vi "monitor.vi"() -> ()   [LabVIEW 2020]
panel:
  out "data_out":dbl[](array[numeric])
  out "controlled_end_point":bool
  in  "heading":dbl format="%.1f"
  in  "y":dbl=383827.29999999877 format="%.1f"
  in  "x":dbl=187655.50000000032 format="%.1f"
  out "XY Graph 2":cluster{"data_out":dbl[], "data_out":dbl[]}[](graph)
  out "endpoint_in_safetyarea":bool
  out "obstacle_in_safetyarea":bool
  out "XY Graph":cluster{"data_out":dbl[], "data_out":dbl[]}[](graph)
  in  "stop":bool
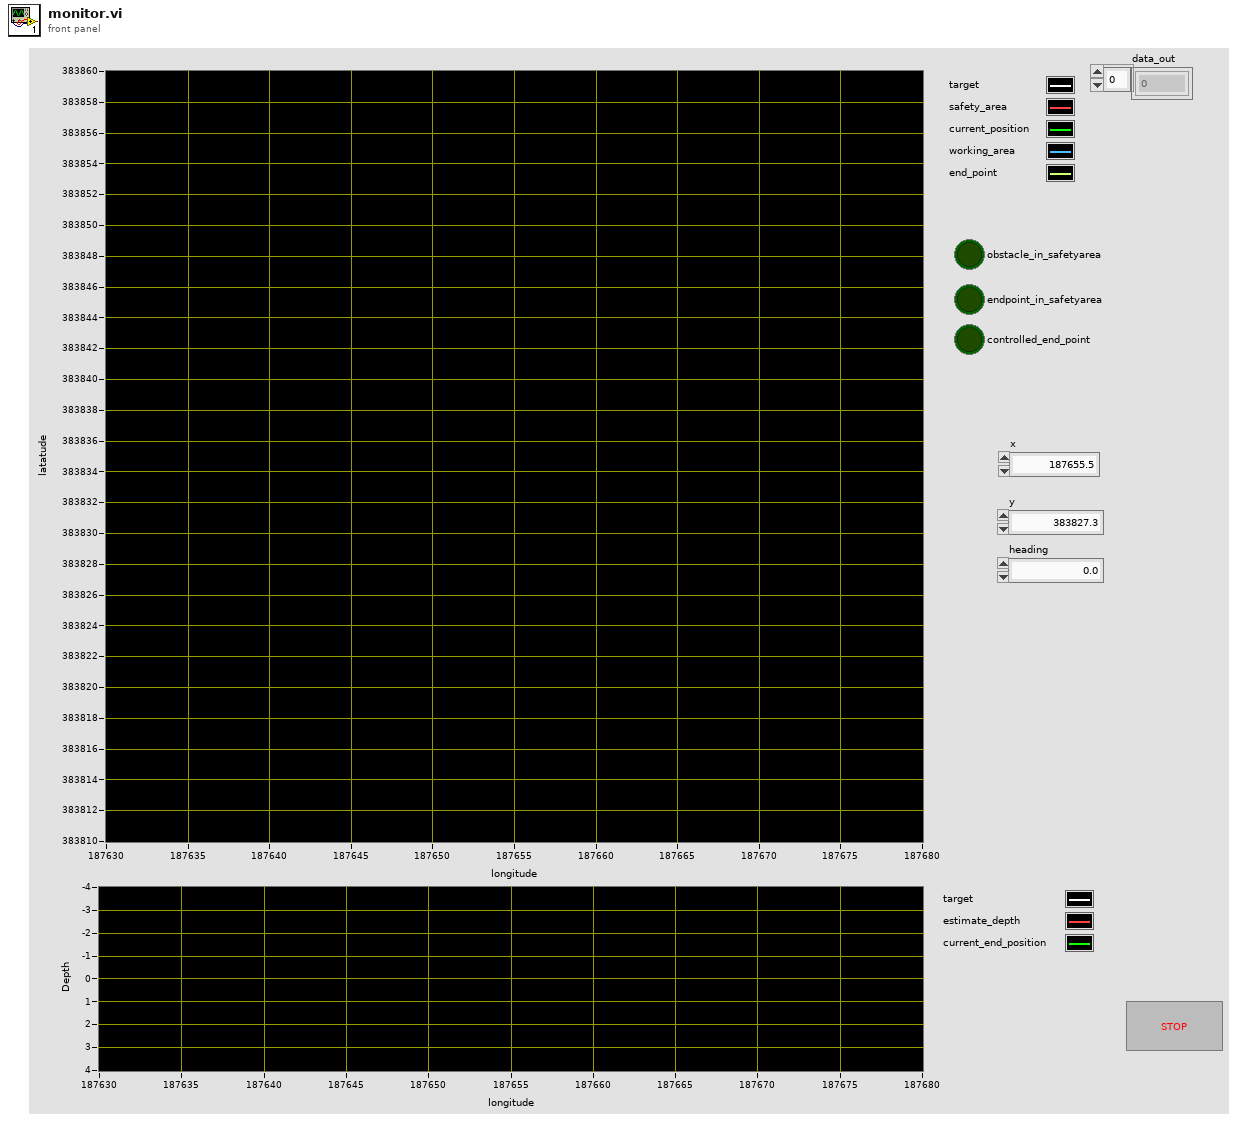
[diagram p1: front panel]
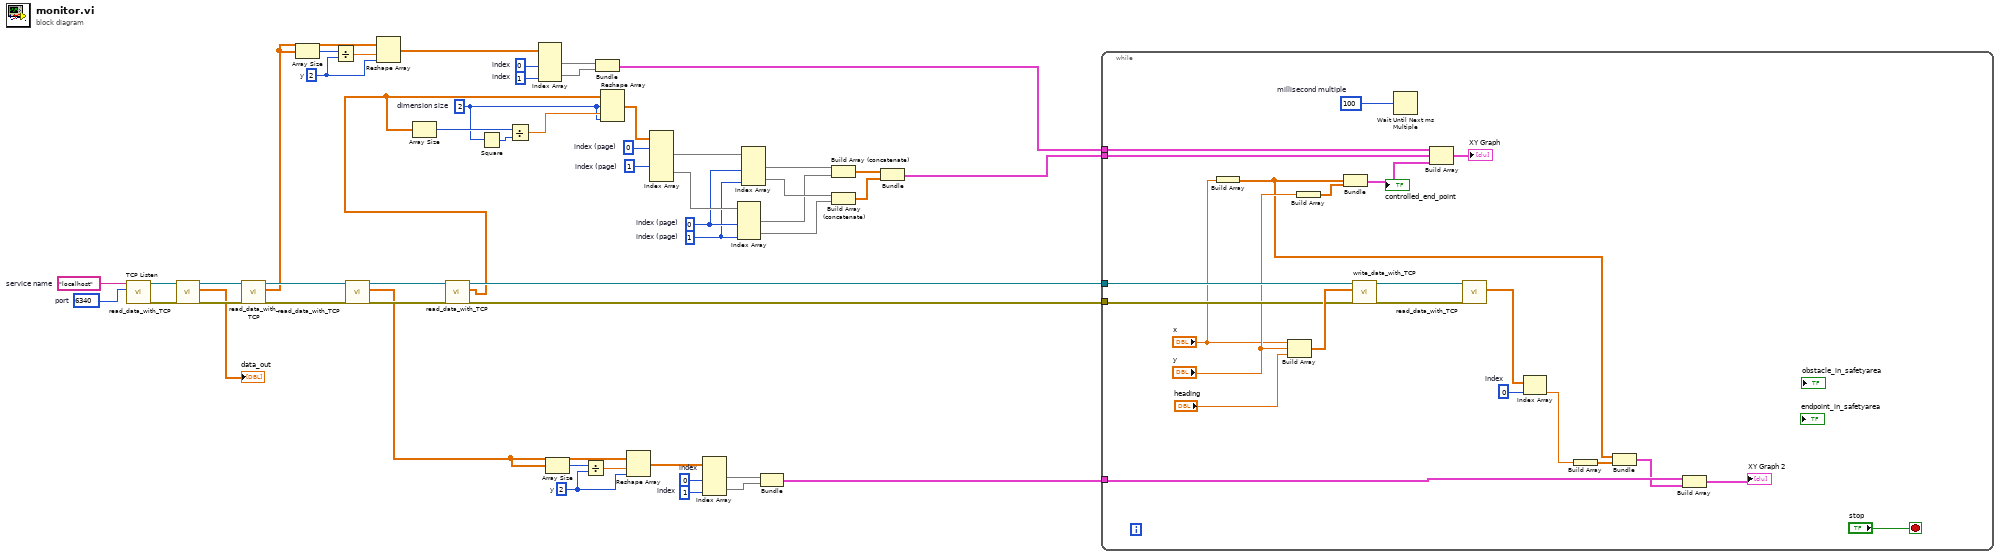
[diagram p0: block diagram]
diagram:
  w19 = 1  # index
  w18 = 0  # index
  w20 = 2  # y
  w25 = 1  # index (page)
  w27 = 1  # index (page)
  w28 = 0  # index (page)
  w26 = 0  # index (page)
  w29 = 2  # dimension size
  w45 = 1  # index
  w46 = 0  # index
  w44 = 2  # y
  w51 = u16 6340  # port
  w52 = "localhost"  # service name
  n1 = call <vilib>:"TCP Listen.vi"("port"=w51, "service name"=w52) -> ("error out"=w3:errorcluster, "connection ID"=w5:refnum<k5>)  [unwired: 5 in, 3 out]
  n2 = call "read_data_with_TCP.vi"("error_in"=w3, "TCP_ref_in"=w5) -> ("error_out"=w2:errorcluster, "data_out"=→"data_out":dbl[], "TCP_ref_out"=w4:refnum<k5>)  [unwired: 7 in]
  n3 = call "read_data_with_TCP.vi"("error_in"=w2, "TCP_ref_in"=w4) -> ("error_out"=w49:errorcluster, "data_out"=w43:dbl[], "TCP_ref_out"=w50:refnum<k5>)  [unwired: 7 in]
  n4 = Array Size(array=w43) -> (size(s)=w47:i32)
  n5 = Divide(x=w47, y=w44) -> (x/y=w48:dbl)
  n6 = call "read_data_with_TCP.vi"("error_in"=w49, "TCP_ref_in"=w50) -> ("error_out"=w14:errorcluster, "data_out"=w7:dbl[], "TCP_ref_out"=w15:refnum<k5>)  [unwired: 7 in]
  n7 = Reshape Array "Reshape Array"(w43, w48, w44) -> (w10:dbl[][])
  n8 = call "read_data_with_TCP.vi"("error_in"=w14, "TCP_ref_in"=w15) -> ("error_out"=w8:errorcluster, "data_out"=w6:dbl[], "TCP_ref_out"=w9:refnum<k5>)  [unwired: 7 in]
  n9 = Array Size(array=w6) -> (size(s)=w32:i32)
  n10 = Square(x=w29) -> (x^2=w33:i32)
  n11 = Divide(x=w32, y=w33) -> (x/y=w34:dbl)
  n12 = Index Array(array=w10, index (col) #1=w46, index (col) #2=w45) -> (element #1=w42:dbl[], element #2=w41:dbl[])  [unwired: 2 in]
  n13 = Array Size(array=w7) -> (size(s)=w17:i32)
  n14 = Divide(x=w17, y=w20) -> (x/y=w16:dbl)
  n15 = Bundle("data_out"=w42, "data_out"=w41) -> (w23:cluster{"data_out":dbl[], "data_out":dbl[]})  [unwired: 1 in]
  n16 = Reshape Array(w6, w29, w34, w29) -> (w30:dbl[][][])
  n17 = Reshape Array "Reshape Array"(w7, w16, w20) -> (w12:dbl[][])
  n18 = Index Array(array=w30, index (dim 0) #1=w26, index (dim 0) #2=w25) -> (element #1=w11:dbl[][], element #2=w31:dbl[][])  [unwired: 4 in]
  n19 = Index Array(array=w12, index (col) #1=w18, index (col) #2=w19) -> (element #1=w21:dbl[], element #2=w22:dbl[])  [unwired: 2 in]
  n20 = Index Array(array=w31, index (col) #1=w28, index (col) #2=w27) -> (element #1=w36:dbl[], element #2=w39:dbl[])  [unwired: 2 in]
  n21 = Index Array(array=w11, index (col) #1=w28, index (col) #2=w27) -> (element #1=w35:dbl[], element #2=w38:dbl[])  [unwired: 2 in]
  n22 = Bundle("data_out"=w21, "data_out"=w22) -> (w13:cluster{"data_out":dbl[], "data_out":dbl[]})  [unwired: 1 in]
  n23 = Build Array (concatenate)(w35, w36) -> (w37:dbl[])
  n24 = Build Array (concatenate)(w38, w39) -> (w40:dbl[])
  n25 = Bundle(w37, w40) -> (w24:cluster{dbl[], dbl[]})  [unwired: 1 in]
  n26 = while {
    tunnel: w24 -> [w72]
    tunnel: w23 -> [w73]
    tunnel: w13 -> [w61]
    tunnel: w9 -> [w70]
    tunnel: w8 -> [w69]
    stop <- "stop" stop-if-true
    w59 = 0  # index
    w68 = u32 100  # millisecond multiple
    n27 = Build Array("x") -> (w55:dbl[])
    n28 = Build Array("x", "y", "heading") -> (w71:dbl[])
    n29 = Build Array("y") -> (w63:dbl[])
    n30 = Bundle(w55, w63) -> (w62:cluster{dbl[], dbl[]})  [unwired: 1 in]
    n31 = call "write_data_with_TCP.vi"("error_in"=w69, "data_in"=w71, "TCP_ref_in"=w70) -> ("error_out"=w65:errorcluster, "TCP_ref_out"=w66:refnum<k5>)  [unwired: 7 in]
    n32 = Wait Until Next ms Multiple(millisecond multiple=w68) -> ()  [unwired: 1 out]
    n33 = Build Array(w73, w72, w62) -> (→"XY Graph":cluster{"data_out":dbl[], "data_out":dbl[]}[])
    n34 = call "read_data_with_TCP.vi"("error_in"=w65, "TCP_ref_in"=w66) -> ("data_out"=w60:dbl[])  [unwired: 7 in, 2 out]
    n35 = Index Array(array=w60, index=w59) -> (element=w57:dbl)
    n36 = Build Array(w57) -> (w56:dbl[])
    n37 = Bundle(w55, w56) -> (w54:cluster{dbl[], dbl[]})  [unwired: 1 in]
    n38 = Build Array(w61, w54) -> (→"XY Graph 2":cluster{"data_out":dbl[], "data_out":dbl[]}[])
  }
